vi "Autonomous Independent.vi"() -> ()   [LabVIEW 2012]
doc: "This VI is called when autonomous begins, and will automatically be terminated when autonomous ends. You can carry out timed or sensor driven robot movement independently without needing to return to the caller."
uses:
  <vilib>/Rock Robotics/WPI/DriverStation/WPI_DriverStationDerivedRobotMode.ctl
  <vilib>/Rock Robotics/WPI/DriverStation/WPI_DriverStationMatch Info.ctl
  Robot Global Data.vi
  <vilib>/Rock Robotics/WPI/Solenoid/Deprecated/WPI_SolenoidSetBool.vi
  <vilib>/addons/control/pid/NI_PID_pid.lvlib
  <vilib>/addons/control/pid/pid.llb/PID (DBL).vi
panel:
  in  "Holding Force":dbl=0.75
  in  "Desired Speed":dbl=9500.0
  in  "Match Info 2":T1={"Autonomous Elapsed Seconds"=0.0, "TeleOp Elapsed Seconds"=0.0, "Disabled Elapsed Seconds"=0.0, "Visited Autonomous"=FALSE, "Visited TeleOp"=FALSE, "Visited Disabled"=FALSE, "Autonomous Settings"={"Autonomous Style"=enum."Independent", "VI Refnum"=refnum}}
  in  "Call Context 2":T2
  # "Be sure to right-click and choose Data Operations>>Make Current Value default if you want to save the array values with the VI"
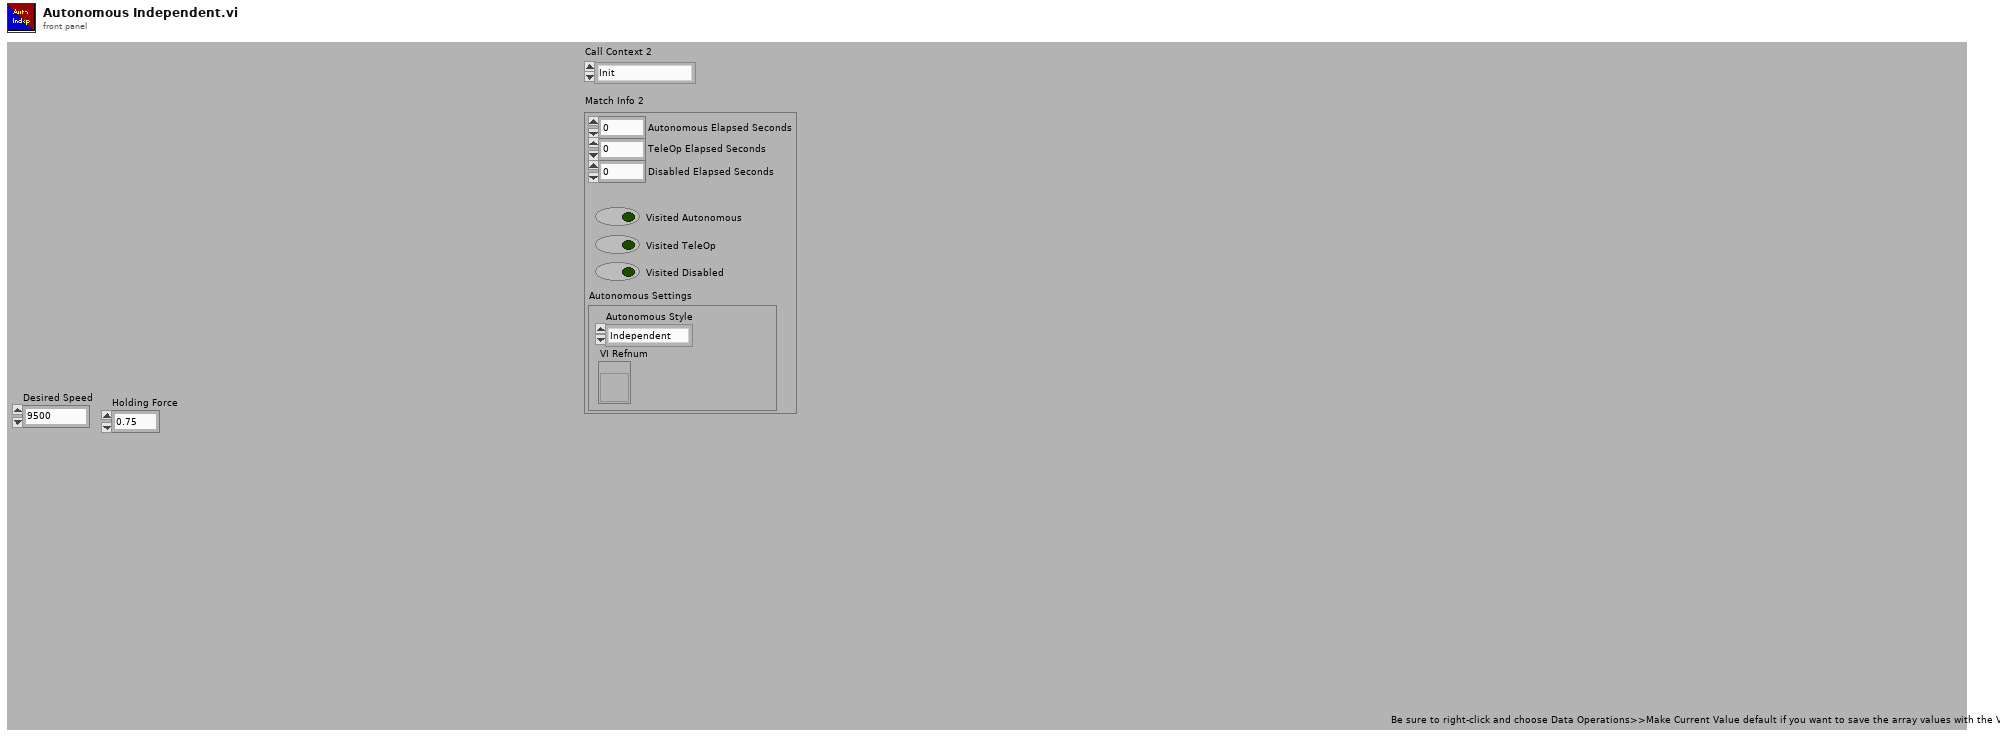
[diagram p1: front panel]
types:
  T1 = typedef "WPI_DriverStationMatch Info.ctl" = cluster{"Autonomous Elapsed Seconds":dbl, "TeleOp Elapsed Seconds":dbl, "Disabled Elapsed Seconds":dbl, "Visited Autonomous":bool, "Visited TeleOp":bool, "Visited Disabled":bool, "Autonomous Settings":cluster{"Autonomous Style":enum16{"Iterative", "Independent"}, "VI Refnum":refnum<vi>}}
  T2 = typedef "WPI_DriverStationDerivedRobotMode.ctl" = enum16{"Init", "Execute", "Stop"}
  T3 = typedef "WPI_SolenoidDevRef.ctl" = cluster{"DevStatus":errorcluster, "Solenoid Module":T4, "Forward Solenoid Channel":T5, "Reverse Solenoid Channel":T5}
  T4 = typedef "FPGA_TypedefSolenoidModule.ctl" = enum16{"Solenoid Module 1", "Solenoid Module 2"}
  T5 = typedef "WPI_SolenoidChannel.ctl" = enum8{"Solenoid 1", "Solenoid 2", "Solenoid 3", "Solenoid 4", "Solenoid 5", "Solenoid 6", "Solenoid 7", "Solenoid 8", "Invalid"}
  T6 = typedef "WPI_MotorControlDeviceRef.ctl" = cluster{"DeviceStatus":errorcluster, "Type":enum16{"PWM", "CAN"}, "PWM":cluster{"Digital Module":T7, "PWM Channel":T8, "DeadBand":T9}, "CAN":cluster{"Device Number":u8, "Control Mode":T10, "Semaphore":T11, "Max Vout":dbl}, "Invert":bool, "TransformRef":T12, "InvTransformRef":T12}
  T7 = typedef "FPGA_TypedefDigitalModule.ctl" = enum16{"Digital Module 1", "Digital Module 2"}
  T8 = typedef "FPGA_DIOPWMChannel.ctl" = enum8{"PWM 1", "PWM 2", "PWM 3", "PWM 4", "PWM 5", "PWM 6", "PWM 7", "PWM 8", "PWM 9", "PWM 10", "Invalid"}
  T9 = typedef "WPI_PWMDeadband.ctl" = cluster{"Name":string, "maxPositivePwm":i32, "minPositivePwm":i32, "centerPwm":i32, "maxNegativePwm":i32, "minNegativePwm":i32, "angularRange":u16}
  T10 = typedef "WPI_CANJaguar_ControlMode.ctl" = enum8{"Percent VBus", "Current", "Speed", "Position", "Voltage"}
  T11 = typedef "Semaphore RefNum" = refnum<k1>
  T12 = typedef "WPI_PWMTransform_ConPane.ctl" = refnum<vi>
  T13 = typedef "WPI_DigitalInputDevRef.ctl" = cluster{"DevStatus":errorcluster, "DIO Channel":T14, "Digital Module":T7}
  T14 = typedef "FPGA_DIOChannel.ctl" = enum8{"DIO 1", "DIO 2", "DIO 3", "DIO 4", "DIO 5", "DIO 6", "DIO 7", "DIO 8", "DIO 9", "DIO 10", "DIO 11", "DIO 12", "DIO 13", "DIO 14", "Invalid"}
  T15 = cluster{"proportional gain (Kc)":dbl, "integral time (Ti, min)":dbl, "derivative time (Td, min)":dbl}
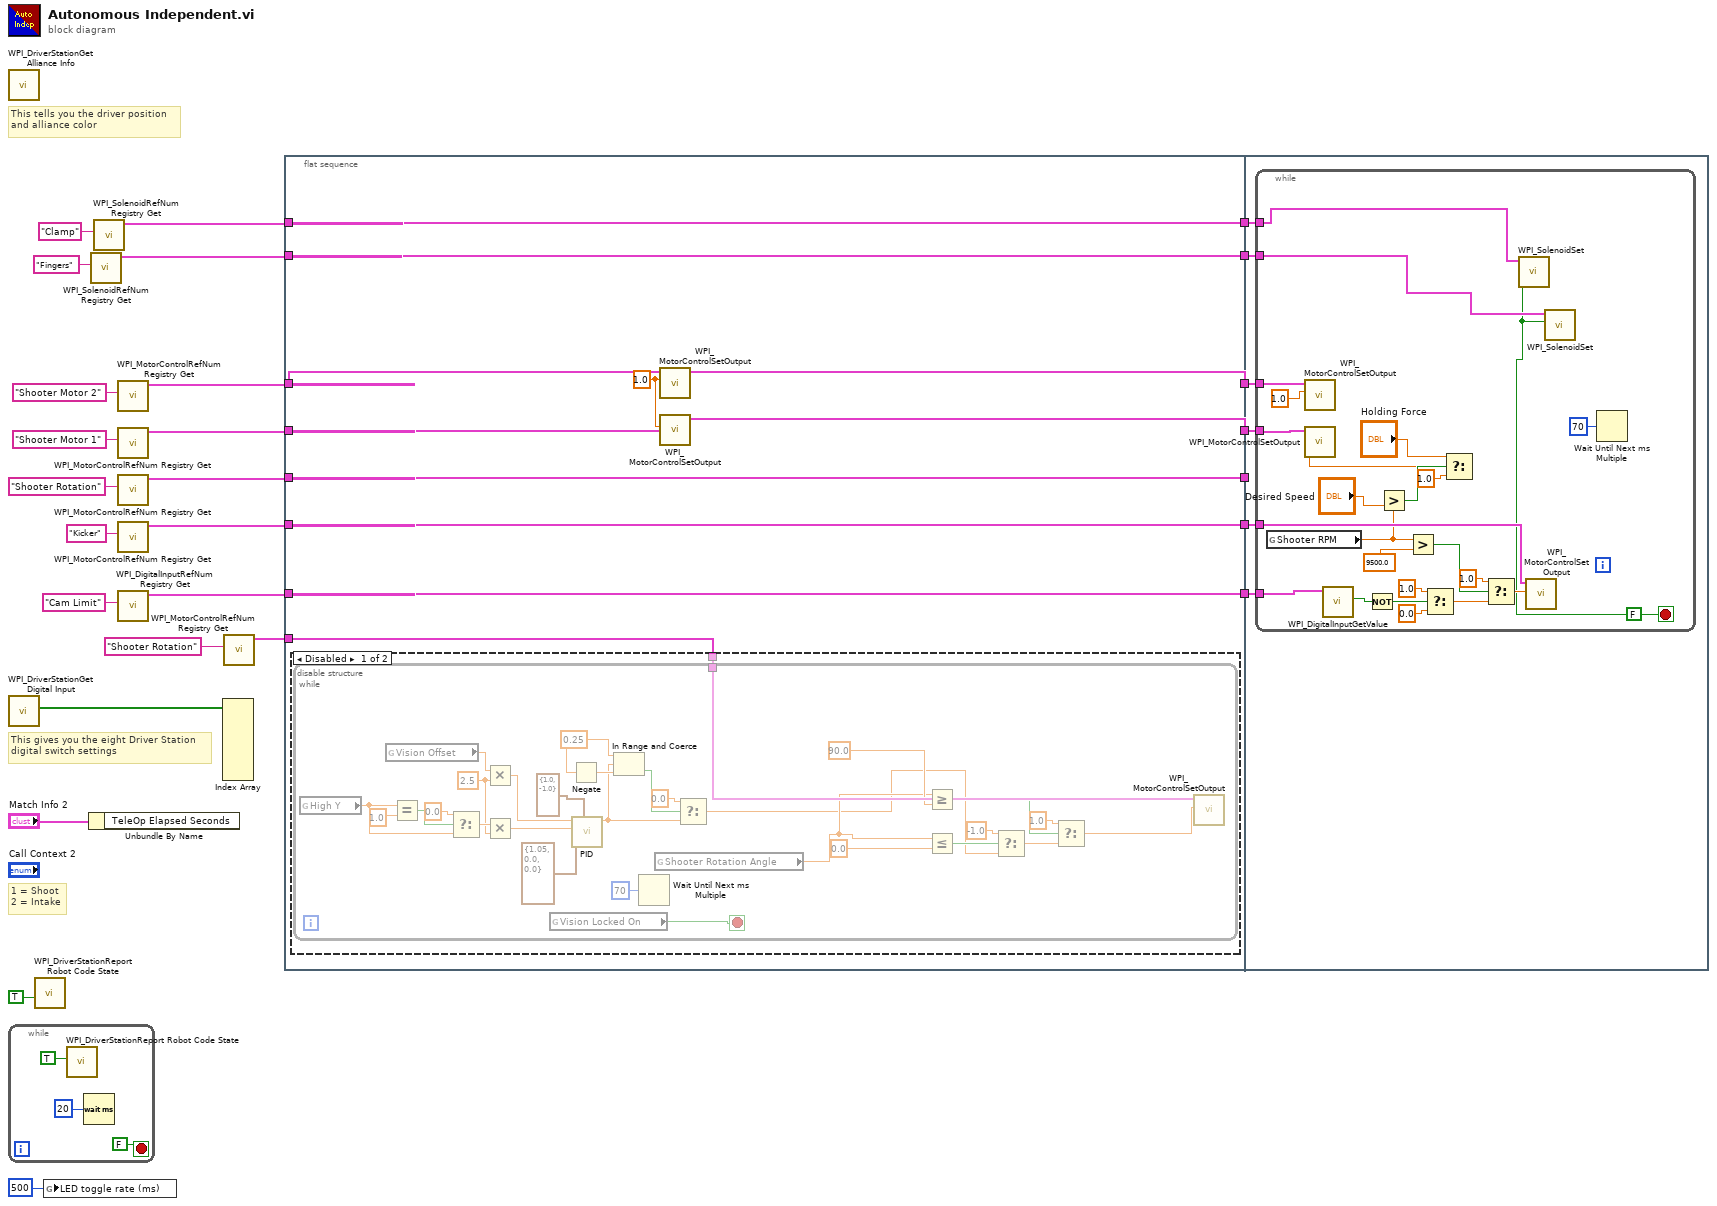
[diagram p0: block diagram]
diagram:
  # "1 = Shoot\n2 = Intake"
  # "This tells you the driver position\nand alliance color"
  # "This gives you the eight Driver Station\ndigital switch settings"
  n1 = call <vilib>:"WPI_DriverStationGet Alliance Info.vi"() -> ()  [unwired: 12 out]
  n2 = call <vilib>:"WPI_DriverStationGet Digital Input.vi"() -> ("Driver Station Digital Input (1-8)"=w17:bool[])  [unwired: 11 out]
  n3 = while {
    stop <- FALSE stop-if-true
    n4 = call <vilib>:"WPI_DriverStationReport Robot Code State.vi"("Autonomous"=TRUE) -> ()  [unwired: 10 in, 1 out]
    n5 = Wait (ms)(milliseconds to wait=u32 20) -> ()  [unwired: 1 out]
  }
  n6 = call <vilib>:"WPI_DriverStationReport Robot Code State.vi"("TeleOp"=TRUE ("Autonomous")) -> ()  [unwired: 10 in, 1 out]
  n7 = global write "Robot Global Data.vi" "LED toggle rate (ms)"(u32 500 ("LED ms toggle rate")) -> ()
  n8 = Unbundle By Name("Match Info 2") -> ()  [unwired: 1 out]
  n9 = call <vilib>:"WPI_SolenoidRefNum Registry Get.vi"("refnum name"="Fingers") -> ("SolenoidDevRef"=w10:T3)  [unwired: 9 in, 1 out]
  n10 = call <vilib>:"WPI_SolenoidRefNum Registry Get.vi"("refnum name"="Clamp") -> ("SolenoidDevRef"=w11:T3)  [unwired: 9 in, 1 out]
  n11 = call <vilib>:"WPI_MotorControlRefNum Registry Get.vi"("refnum name"="Shooter Motor 2") -> ("MotorControlDevRef"=w18:T6)  [unwired: 9 in, 1 out]
  n12 = call <vilib>:"WPI_MotorControlRefNum Registry Get.vi"("refnum name"="Shooter Motor 1") -> ("MotorControlDevRef"=w19:T6)  [unwired: 9 in, 1 out]
  n13 = call <vilib>:"WPI_MotorControlRefNum Registry Get.vi"("refnum name"="Shooter Rotation") -> ("MotorControlDevRef"=w20:T6)  [unwired: 9 in, 1 out]
  n14 = call <vilib>:"WPI_MotorControlRefNum Registry Get.vi"("refnum name"="Kicker") -> ("MotorControlDevRef"=w16:T6)  [unwired: 9 in, 1 out]
  n15 = call <vilib>:"WPI_DigitalInputRefNum Registry Get.vi"("refnum name"="Cam Limit") -> ("DigitalInputDevRef"=w14:T13)  [unwired: 9 in, 1 out]
  n16 = Index Array(array=w17) -> ()  [unwired: 8 in, 8 out]
  n17 = call <vilib>:"WPI_MotorControlRefNum Registry Get.vi"("refnum name"="Shooter Rotation") -> ("MotorControlDevRef"=w8:T6)  [unwired: 9 in, 1 out]
  n18 = flat-sequence {
    tunnel: w10 -> [w37]
    tunnel: w11 -> [w38]
    tunnel: w14 -> [w39]
    tunnel: w16 -> [w40]
    tunnel: w18 -> [w32]
    tunnel: w19 -> [w35]
    tunnel: w20 -> [w41]
    tunnel: [w41] -> w7
    tunnel: [w34] -> w6
    tunnel: [w33] -> w5
    tunnel: [w40] -> w4
    tunnel: [w39] -> w3
    tunnel: [w38] -> w2
    tunnel: [w37] -> w1
    tunnel: w8 -> [w36]
    tunnel: w7 -> [_]
    tunnel: w6 -> [w76]
    tunnel: w5 -> [w75]
    tunnel: w4 -> [w77]
    tunnel: w3 -> [w74]
    tunnel: w2 -> [w73]
    tunnel: w1 -> [w72]
    frame #0 {
      w31 = 1.0 ("Output")
      n19 = disable-structure shown="Disabled" {
        disable-tunnel: w36 -> [w42 _]
        frame Disabled {
          n20 = while {
            tunnel: w42 -> [w57]
            stop <- w53 stop-if-true
            w70 = 0.25 ("x")
            w63 = 2.5 ("y")
            n21 = global read "Robot Global Data.vi" "High Y"() -> (w58:dbl)
            n22 = global read "Robot Global Data.vi" "Vision Offset"() -> (w60:dbl)
            n23 = Equal?(x=w58, y=1.0) -> (x = y?=w59:bool)
            n24 = Select(t=0.0, s=w59, f=w58) -> (s? t:f=w64:dbl)
            n25 = Multiply(x=w60, y=w63) -> (x*y=w62:dbl)
            n26 = Multiply(x=w64, y=w63) -> (x*y=w61:dbl)
            n27 = global read "Robot Global Data.vi" "Vision Locked On"() -> (w53:bool)
            n28 = Negate(x=w70) -> (-x=w71:dbl)
            n29 = call-poly <vilib>:"PID.vi"("output range"=cluster{"output high":dbl, "output low":dbl} {"output high"=1.0, "output low"=-1.0}, "PID gains"=T15 {"proportional gain (Kc)"=1.05, "integral time (Ti, min)"=0.0, "derivative time (Td, min)"=0.0}, "process variable"=w61, "setpoint"=w62) -> ("output"=w68:dbl)  [unwired: 6 in, 1 out]
            n30 = In Range and Coerce(upper limit=w70, x=w68, lower limit=w71) -> (In Range?=w55:bool)  [unwired: 1 out]
            n31 = Wait Until Next ms Multiple(millisecond multiple=u32 70) -> ()  [unwired: 1 out]
            n32 = global read "Robot Global Data.vi" "Shooter Rotation Angle"() -> (w45:dbl)
            n33 = Select(t=0.0, s=w55, f=w68) -> (s? t:f=w44:dbl)
            n34 = Greater Or Equal?(x=w45, y=90.0 ("upper limit")) -> (x >= y?=w47:bool)
            n35 = Less Or Equal?(x=w45, y=0.0 ("lower limit")) -> (x <= y?=w48:bool)
            n36 = Select(t=-1.0, s=w48, f=w44) -> (s? t:f=w52:dbl)
            n37 = Select(t=1.0, s=w47, f=w52) -> (s? t:f=w43:dbl)
            n38 = call <vilib>:"WPI_MotorControlSetOutput.vi"("Output"=w43, "MotorControlDevRef"=w57) -> ()  [unwired: 7 in, 3 out]
          }
        }
        frame Enabled {
        }
      }
      n39 = call <vilib>:"WPI_MotorControlSetOutput.vi"("Output"=w31, "MotorControlDevRef"=w32) -> ("MotorControlDevRef"=w33:T6)  [unwired: 7 in, 2 out]
      n40 = call <vilib>:"WPI_MotorControlSetOutput.vi"("Output"=w31, "MotorControlDevRef"=w35) -> ("MotorControlDevRef"=w34:T6)  [unwired: 7 in, 2 out]
    }
    frame #1 {
      n41 = while {
        tunnel: w77 -> [w94]
        tunnel: w76 -> [w93]
        tunnel: w75 -> [w92]
        tunnel: w74 -> [w88]
        tunnel: w73 -> [w86]
        tunnel: w72 -> [w85]
        stop <- w78 stop-if-true
        w78 = FALSE
        n42 = global read "Robot Global Data.vi" "Shooter RPM"() -> (w80:dbl)
        n43 = call <vilib>:"WPI_MotorControlSetOutput.vi"("Output"=1.0, "MotorControlDevRef"=w92) -> ()  [unwired: 7 in, 3 out]
        n44 = call <vilib>:"WPI_DigitalInputGetValue.vi"("DigitalInputDevRef"=w88) -> ("Value"=w99:bool)  [unwired: 8 in, 2 out]
        n45 = Not(x=w99) -> (.not. x?=w98:bool)
        n46 = Greater?(x=w80, y="Desired Speed") -> (0:w83:bool)
        n47 = Greater?(x=w80, y=9500.0 ("Minimum Speed")) -> (0:w100:bool)
        n48 = Select(t=1.0, s=w98, f=0.0) -> (s? t:f=w97:dbl)
        n49 = Select(t="Holding Force", s=w83, f=1.0 ("Shooter Speed")) -> (s? t:f=w79:dbl)
        n50 = call <vilib>:"WPI_MotorControlSetOutput.vi"("Output"=w79, "MotorControlDevRef"=w93) -> ()  [unwired: 7 in, 3 out]
        n51 = Select(t=1.0, s=w100, f=w97) -> (s? t:f=w89:dbl)
        n52 = call-poly <vilib>:"WPI_SolenoidSet.vi"("Value"=w78, "SolenoidDevRef"=w86) -> ()  [unwired: 8 in, 2 out]
        n53 = call <vilib>:"WPI_MotorControlSetOutput.vi"("Output"=w89, "MotorControlDevRef"=w94) -> ()  [unwired: 7 in, 3 out]
        n54 = call-poly <vilib>:"WPI_SolenoidSet.vi"("Value"=w78, "SolenoidDevRef"=w85) -> ()  [unwired: 8 in, 2 out]
        n55 = Wait Until Next ms Multiple(millisecond multiple=u32 70) -> ()  [unwired: 1 out]
      }
    }
  }
